vi "GDSString_PatternMatching.vi"(0 "TextIn":string, 1 "PatternMatchingStrings":string[](array[string]), 2 "StringStartOffset(Default=-1 => 0 for Forward, StrLenght for Backwards)":i32=-1, 3 "Search Backwards":bool, 5 "error in (no error)":errorcluster, 6 "IgnoreMatchesWithinThesePositions":i32[][](array[numeric])) -> (13 "IndexOfTheFoundPatternMatchingString":i32=1, 14 "TextBefore":string, 15 "Match":string, 16 "TextAfter":string, 17 "IndexAfterMatch(Or before when searching Backwards)":i32=1, 18 "Found":bool, 19 "error out":errorcluster)   [LabVIEW 2012]
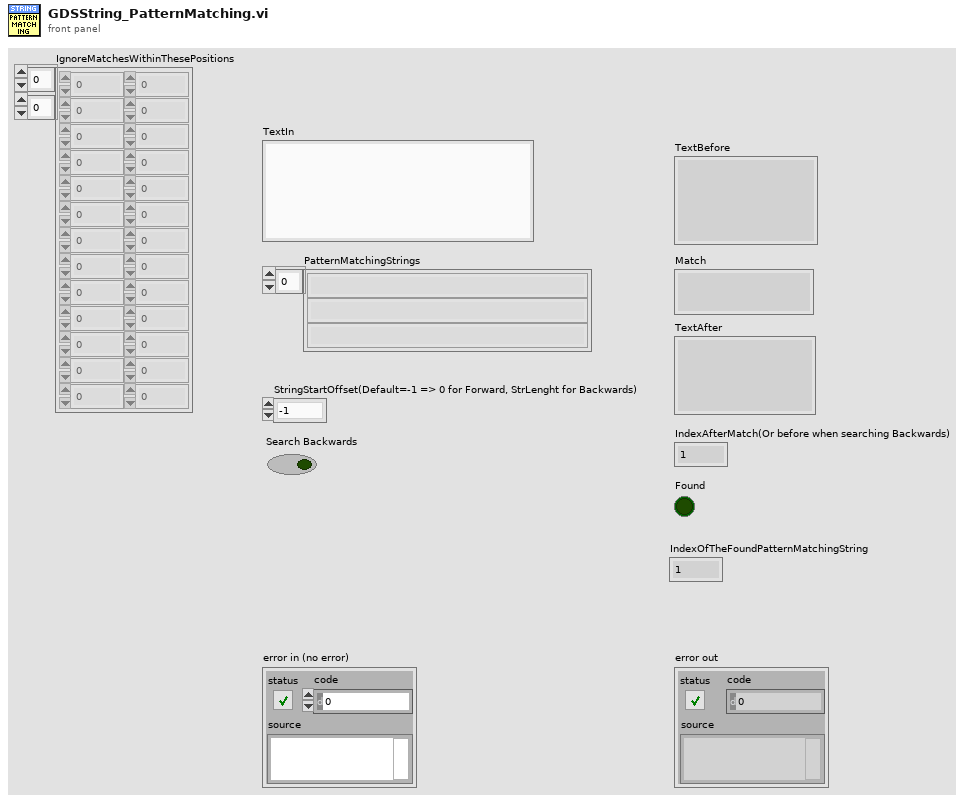
[diagram p1: front panel]
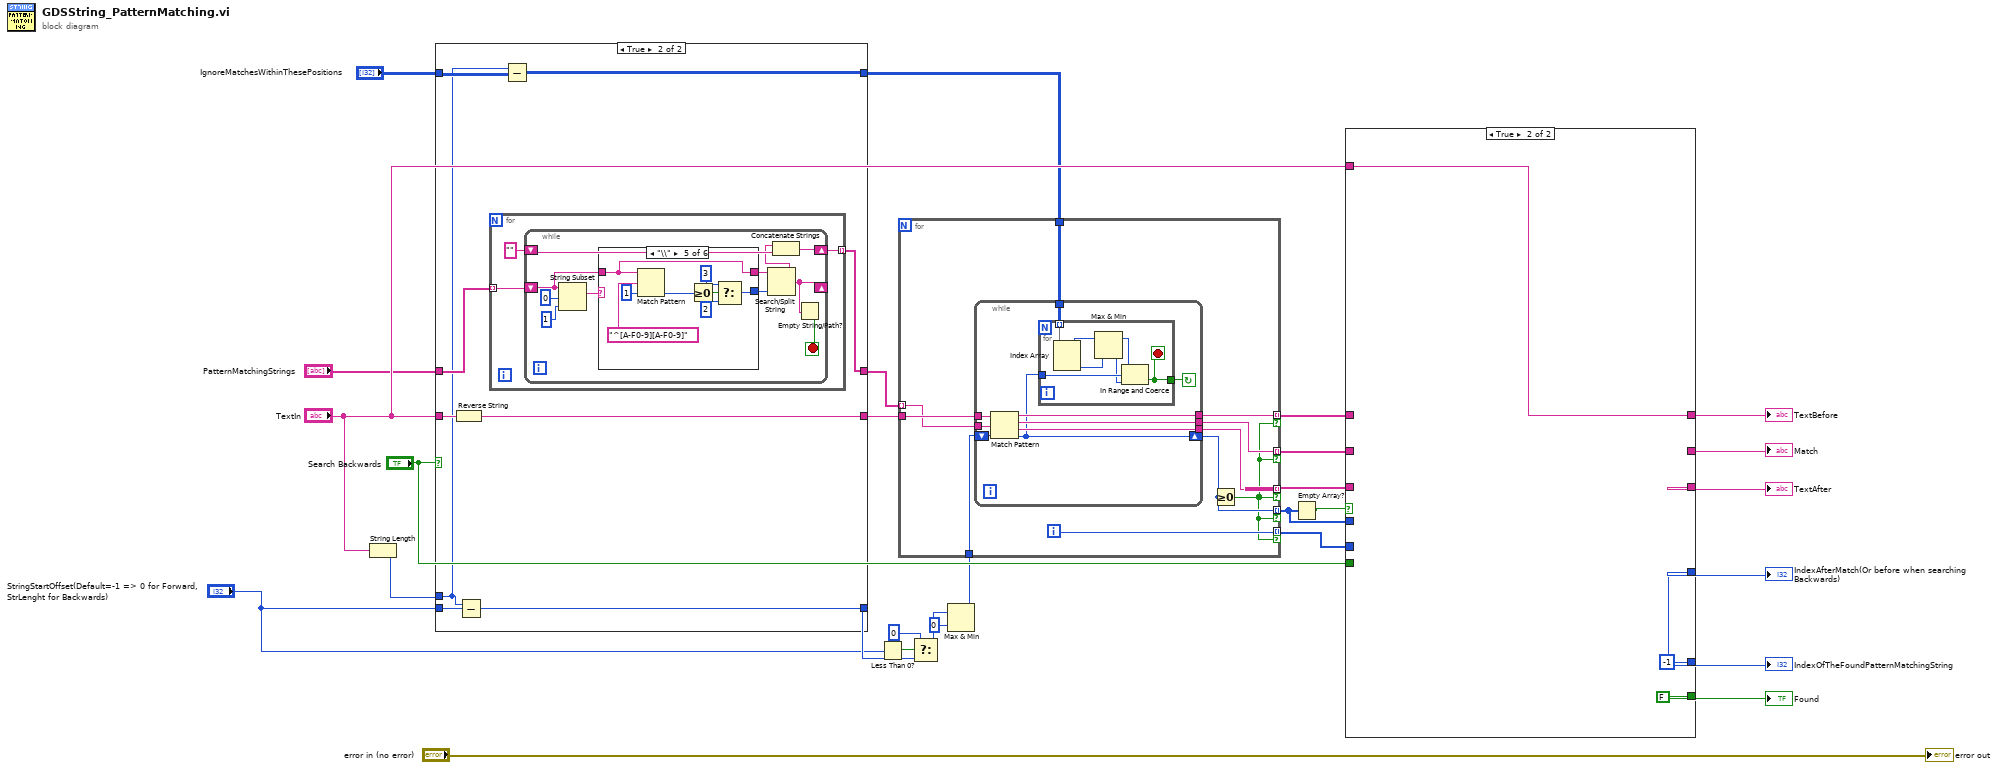
[diagram p0: block diagram]
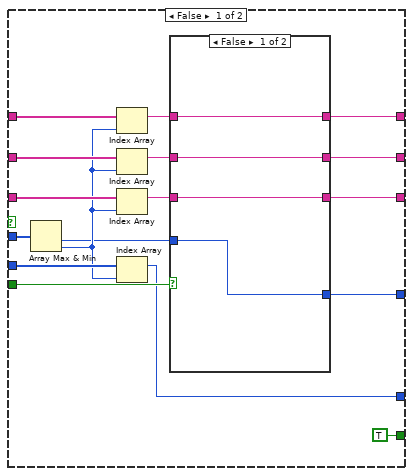
[diagram p2: hidden frame]
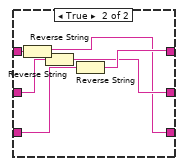
[diagram p3: hidden frame]
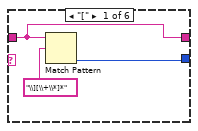
[diagram p5: hidden frame]
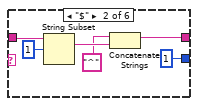
[diagram p6: hidden frame]
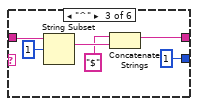
[diagram p7: hidden frame]
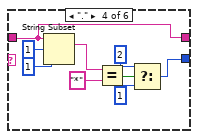
[diagram p8: hidden frame]
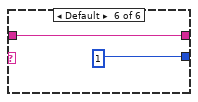
[diagram p9: hidden frame]
diagram:
  n1 = String Length(string="TextIn") -> (length=w13:i32)
  n2 = case shown="True" "Search Backwards" {
    tunnel: [w32 w41] -> w26
    tunnel: "TextIn" -> [w32 w40]
    tunnel: "StringStartOffset(Default=-1 => 0 for Forward, StrLenght for Backwards)" -> [w31 w38]
    tunnel: [w31 w39] -> w7
    tunnel: w13 -> [_ w34]
    tunnel: "PatternMatchingStrings" -> [w30 w37]
    tunnel: [w30 w36] -> w3
    tunnel: "IgnoreMatchesWithinThesePositions" -> [w29 w35]
    tunnel: [w29 w33] -> w1
    frame False {
    }
    frame True {
      n3 = Reverse String(1:w40) -> (0:w41:string)
      n4 = Subtract(x=w34, y=w38) -> (x-y=w39:i32)
      n5 = for {
        tunnel: w37 -> [w44] mode=indexing
        tunnel: [w42] -> w36 mode=indexing
        n6 = while {
          shift-right: [w48] -> _
          shift-left: w44 -> [w46]
          shift-right: [w52] -> w42
          shift-left: "" -> [w51]
          stop <- w47 stop-if-true
          n7 = String Subset(string=w46, offset (0)=0, length (rest)=1 ("length (rest)")) -> (substring=w53:string)
          n8 = case shown="\"\\\\\"" w53 {
            tunnel: [w57 1 ("offset (0)") 1 ("offset (0)") w72 w81 1 ("offset (0)")] -> w50
            tunnel: w46 -> [w56 w64 w70 w71 w80 w88]
            tunnel: [w56 w60 w66 w71 w80 w88] -> w45
            frame "[" {
              n9 = Match Pattern(string=w56, regular expression="\\][\\+\\*]*") -> (offset past match=w57:i32)  [unwired: 1 in, 3 out]
            }
            frame "$" {
              n10 = String Subset(string=w64, offset (0)=1) -> (substring=w62:string)  [unwired: 1 in]
              n11 = Concatenate Strings("^" ("regular expression"), w62) -> (w60:string)
            }
            frame "^" {
              n12 = String Subset(string=w70, offset (0)=1) -> (substring=w68:string)  [unwired: 1 in]
              n13 = Concatenate Strings("$" ("regular expression"), w68) -> (w66:string)
            }
            frame "." {
              n14 = String Subset(string=w71, offset (0)=1, length (rest)=1 ("length (rest)")) -> (substring=w77:string)
              n15 = Equal?(x=w77, y="*") -> (x = y?=w73:bool)
              n16 = Select(t=2 ("x"), s=w73, f=1 ("x")) -> (s? t:f=w72:i32)
            }
            frame "\\" {
              n17 = Match Pattern(string=w80, regular expression="^[A-F0-9][A-F0-9]", offset (0)=1) -> (offset past match=w86:i32)  [unwired: 3 out]
              n18 = Greater Or Equal To 0?(x=w86) -> (x >= 0?=w85:bool)
              n19 = Select(t=3 ("x"), s=w85, f=2 ("x")) -> (s? t:f=w81:i32)
            }
            frame Default {
            }
          }
          n20 = Search/Split String(string=w45, offset (0)=w50) -> (substring before match=w49:string, match + rest of string=w48:string)  [unwired: 1 in, 1 out]
          n21 = Concatenate Strings(w49, w51) -> (w52:string)
          n22 = Empty String/Path?(string/path=w48) -> (empty?=w47:bool)
        }
      }
      n23 = Subtract(x=w34, y=w35) -> (x-y=w33:i32[][])
    }
  }
  n24 = Less Than 0?(x="StringStartOffset(Default=-1 => 0 for Forward, StrLenght for Backwards)") -> (x < 0?=w9:bool)
  n25 = Select(t=0, s=w9, f=w7) -> (s? t:f=w8:i32)
  n26 = Max & Min(x=w8, y=0) -> (max(x,y)=w12:i32)  [unwired: 1 out]
  n27 = for {
    tunnel: w26 -> [w99]
    tunnel: [w98] -> w27 mode=indexing if=w91
    tunnel: [w97] -> w28 mode=indexing if=w91
    tunnel: w3 -> [w96] mode=indexing
    tunnel: w12 -> [w95]
    tunnel: [w94] -> w25 mode=indexing if=w91
    tunnel: [w93] -> w17 mode=indexing if=w91
    tunnel: [w92] -> w18 mode=indexing if=w91
    tunnel: w1 -> [w90]
    i -> [w93]
    n28 = while {
      tunnel: w99 -> [w108]
      tunnel: [w107] -> w98
      tunnel: [w106] -> w97
      tunnel: w96 -> [w105]
      tunnel: [w103] -> w94
      shift-right: [w102] -> w92
      shift-left: w95 -> [w104]
      tunnel: w90 -> [w101]
      stop <- w100 continue-if-true
      n29 = Match Pattern(string=w108, regular expression=w105, offset (0)=w104) -> (before substring=w106:string, match substring=w103:string, after substring=w107:string, offset past match=w102:i32)
      n30 = for {
        tunnel: w101 -> [w114] mode=indexing
        tunnel: w102 -> [w115]
        tunnel: [w113] -> w100
        stop <- w113 stop-if-true
        n31 = Index Array(array=w114) -> (element #1=w112:i32, element #2=w111:i32)  [unwired: 2 in]
        n32 = Max & Min(x=w112, y=w111) -> (max(x,y)=w109:i32, min(x,y)=w110:i32)
        n33 = In Range and Coerce(upper limit=w109, x=w115, lower limit=w110) -> (In Range?=w113:bool)  [unwired: 1 out]
      }
    }
    n34 = Greater Or Equal To 0?(x=w92) -> (x >= 0?=w91:bool)
  }
  n35 = Empty Array?(array=w18) -> (empty?=w23:bool)
  n36 = case shown="True" w23 {
    tunnel: w28 -> [w132 _]
    tunnel: w27 -> [w131 _]
    tunnel: w25 -> [w130 _]
    tunnel: "Search Backwards" -> [w129 _]
    tunnel: [TRUE FALSE] -> w21
    tunnel: [w119 w144] -> w20
    tunnel: [w117 w144] -> w19
    tunnel: w18 -> [w128 _]
    tunnel: w17 -> [w127 _]
    tunnel: [w122 w143] -> w16
    tunnel: [w121 _] -> w15
    tunnel: [w120 _] -> w14
    tunnel: "TextIn" -> [_ w143]
    frame False {
      n37 = Array Max & Min(array=w128) -> (min value=w118:i32, min index (indices)=w123:i32)  [unwired: 2 out]
      n38 = Index Array(array=w132, index=w123) -> (element=w124:string)
      n39 = Index Array(array=w130, index=w123) -> (element=w125:string)
      n40 = Index Array(array=w131, index=w123) -> (element=w126:string)
      n41 = Index Array(array=w127, index=w123) -> (element=w119:i32)
      n42 = case shown="False" w129 {
        tunnel: w124 -> [w136 w142]
        tunnel: w126 -> [w134 w141]
        tunnel: w125 -> [w135 w140]
        tunnel: [w136 w139] -> w122
        tunnel: [w135 w138] -> w121
        tunnel: [w134 w137] -> w120
        tunnel: w118 -> [w133 _]
        tunnel: [w133 _] -> w117
        frame False {
        }
        frame True {
          n43 = Reverse String(1:w142) -> (0:w137:string)
          n44 = Reverse String(1:w140) -> (0:w138:string)
          n45 = Reverse String(1:w141) -> (0:w139:string)
        }
      }
    }
    frame True {
      w144 = -1 ("IndexOfmatchStringFound")
    }
  }
  "TextBefore" <- w16
  "Match" <- w15
  "TextAfter" <- w14
  "IndexAfterMatch(Or before when searching Backwards)" <- w19
  "IndexOfTheFoundPatternMatchingString" <- w20
  "Found" <- w21
  "error out" <- "error in (no error)"
